vi "circulo.vi"() -> ()   [LabVIEW 2016]
panel:
  out "XY Graph":cluster{dbl[], dbl[]}(graph)
  out "Waveform Graph":dbl[][](graph)
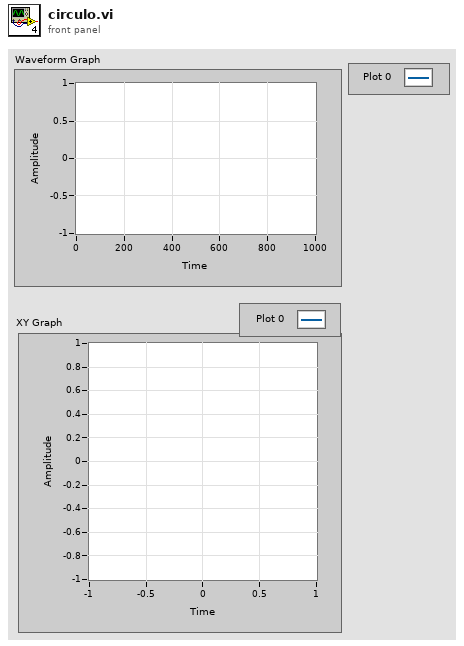
[diagram p1: front panel]
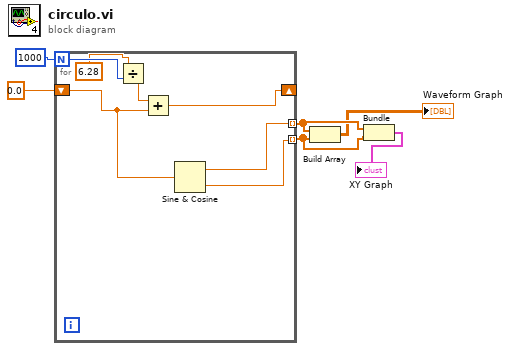
[diagram p0: block diagram]
diagram:
  n1 = for {
    N: 1000 -> [w13]
    shift-right: [w10] -> _
    shift-left: 0.0 -> [w9]
    tunnel: [w8] -> w4 mode=indexing
    tunnel: [w7] -> w3 mode=indexing
    n2 = Divide(x=6.28, y=w13) -> (x/y=w11:dbl)
    n3 = Add(x=w11, y=w9) -> (x+y=w10:dbl)
    n4 = Sine & Cosine(0:w9) -> (1:w8:dbl, 2:w7:dbl)
  }
  n5 = Build Array(w4, w3) -> (→"Waveform Graph":dbl[][])
  n6 = Bundle(w4, w3) -> (→"XY Graph":cluster{dbl[], dbl[]})  [unwired: 1 in]
